vi "ClusterEscala.vi"() -> ()   [LabVIEW 2020]
panel:
  out "Cluster 2":T1 {"Presión" scale=0.0..100.0; "Flujo" scale=0.0..100.0; "Temperatura" scale=0.0..100.0}
  in  "Cluster":T2
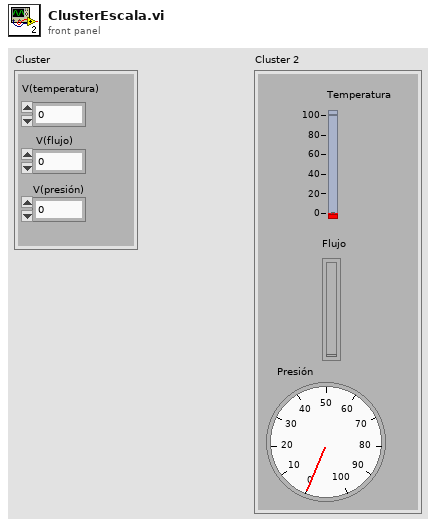
[diagram p1: front panel]
types:
  T1 = cluster{"Temperatura":dbl, "Flujo":u8, "Presión":dbl}
  T2 = cluster{"V(temperatura)":dbl, " V(flujo)":dbl, "V(presión)":dbl}
  T3 = cluster{"C/V":dbl, "(I/seg)/V":dbl, "(N/m^2)/V":dbl}
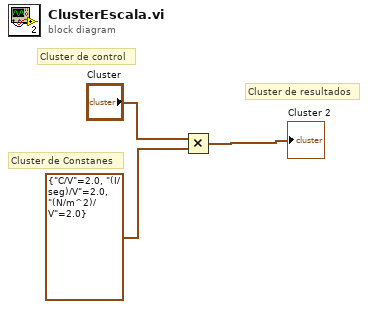
[diagram p0: block diagram]
diagram:
  # "Cluster de resultados"
  # "Cluster de Constanes"
  # "Cluster de control"
  n1 = Multiply(x="Cluster", y=T3 {"C/V"=2.0, "(I/seg)/V"=2.0, "(N/m^2)/V"=2.0}) -> (x*y=→"Cluster 2":cluster{dbl, dbl, dbl})
